vi "DAQEG_DAQ DATA Queue FGV.vi"(6 "Command":enum16{"Initialize", "Get Value", "Set Value"}(ring)=enum."Get Value", 8 "error in (no error)":errorcluster, 11 "DAQ DATA":T1(array[cluster])) -> (0 "error out":errorcluster, 3 "DAQ DATA Out":T1(array[cluster]))   [LabVIEW 2016]
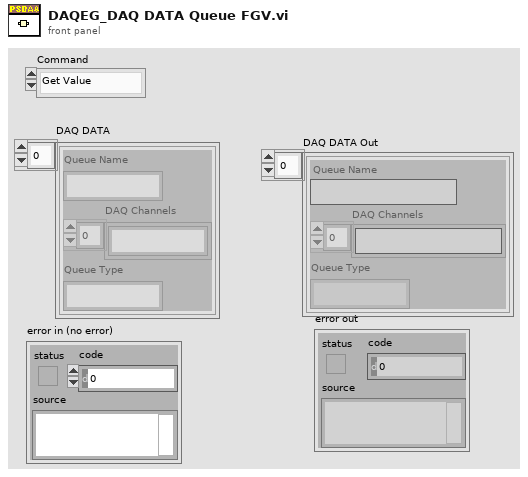
[diagram p1: front panel]
types:
  T1 = cluster{"Queue Name":string, "DAQ Channels":string[], "Queue Type":string}[]
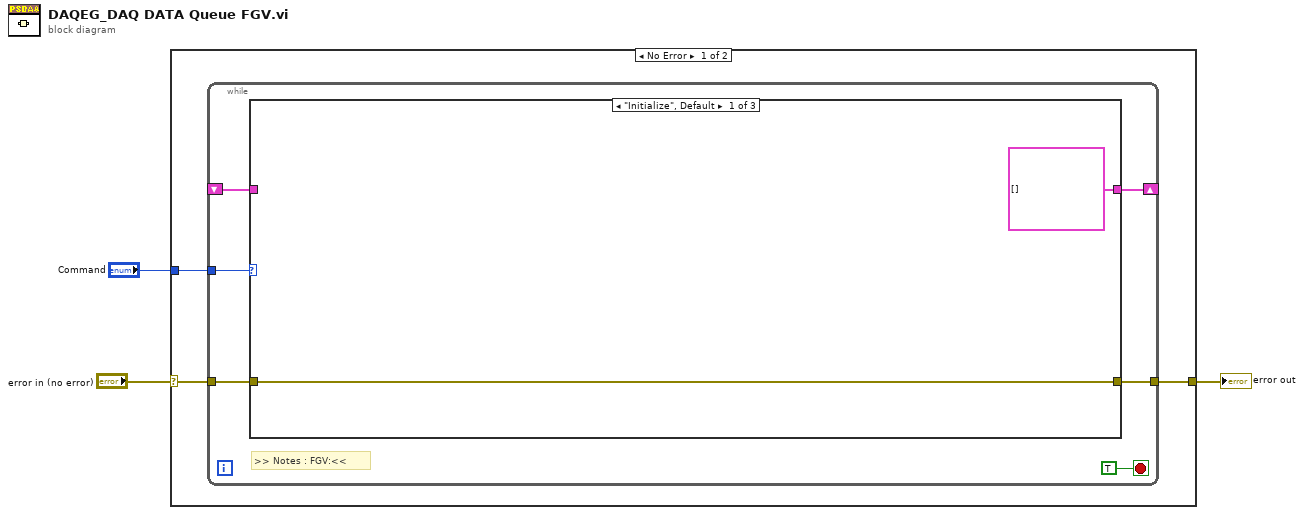
[diagram p0: block diagram]
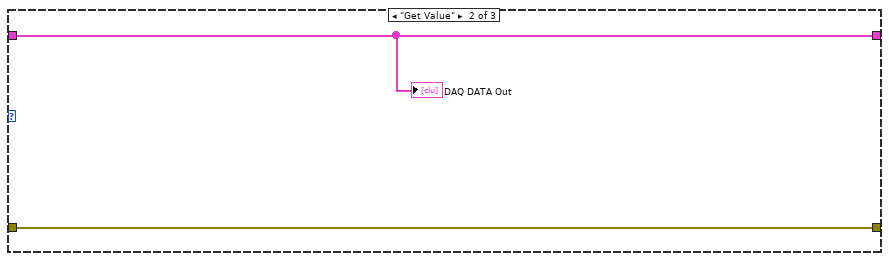
[diagram p2: hidden frame]
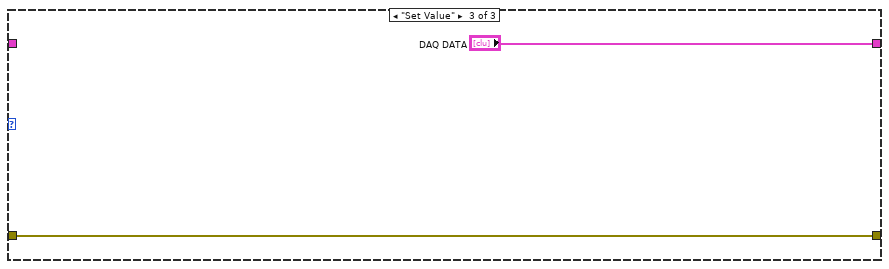
[diagram p3: hidden frame]
diagram:
  n1 = case shown="No Error" "error in (no error)" {
    selector: "error in (no error)" -> [w5 w19]
    tunnel: [w4 w19] -> w3
    tunnel: "Command" -> [w6 _]
    frame No Error {
      n2 = while {
        tunnel: w6 -> [w11]
        tunnel: w5 -> [w10]
        tunnel: [w9] -> w4
        shift-right: [w8] -> _
        shift-left: _ -> [w7]
        stop <- TRUE stop-if-true
        # ">> Notes : FGV:<<"
        n3 = case shown="\"Initialize\", Default" w11 {
          tunnel: w10 -> [w14 w16 w18]
          tunnel: [w14 w16 w18] -> w9
          tunnel: [T1 [] ("DAQ DATA") w15 "DAQ DATA"] -> w8
          tunnel: w7 -> [_ w15 _]
          frame "Initialize", Default {
          }
          frame "Get Value" {
            "DAQ DATA Out" <- w15
          }
          frame "Set Value" {
          }
        }
      }
    }
    frame Error {
    }
  }
  "error out" <- w3
